vi "Stop Core.vi"(10 "final error code":i32, 11 "Iterator Actor in":refnum<class "Iterator Actor.lvclass">) -> (3 "Iterator Actor out":refnum<class "Iterator Actor.lvclass">)   [LabVIEW 2016, in "Iterator Actor.lvlib" / "Iterator Actor.lvclass"]
doc: "(<B>Filename</B>: Actor Framework.lvlib:Actor.lvclass:Stop Core.vi)\n\nDefines what the actor does before it stops. Use the <B>final error code</B> input to determine whether the actor shut down in response to an error.\n\nBy default, this method does nothing. A descendant class may override it to define behavior, such as shutting down any processes the actor initiated in its override of the Actor Core method."
uses:
  Iterator Actor.lvclass
  Iterator Actor.lvclass/Iterator Actor.ctl
  <vilib>/ActorFramework/Actor/Actor.lvclass
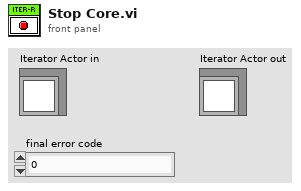
[diagram p1: front panel]
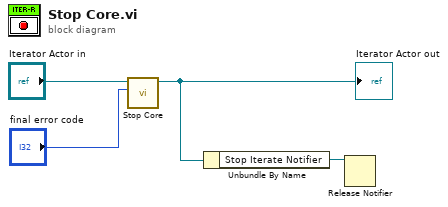
[diagram p0: block diagram]
diagram:
  n1 = call-parent "Stop Core.vi"("final error code"="final error code", "Actor in"="Iterator Actor in") -> ("Actor out"=w1:refnum<class "Iterator Actor.lvclass">)  [unwired: 9 in]
  "Iterator Actor out" <- w1
  n2 = Unbundle By Name(w1) -> ("Stop Iterate Notifier"=w2:refnum<notifier>)
  n3 = Release Notifier(notifier=w2) -> ()  [unwired: 2 in, 3 out]
